vi "ADO Recordset GetString.vi"(0 "ADODB._Recordset":refnum<k7>, 1 "NumRows":i32=-1, 5 "error in (no error)":errorcluster) -> (14 "ADODB._Recordset Out":refnum<k7>, 15 "GetString":string, 19 "error out":errorcluster)   [LabVIEW 2018]
doc: "<FUNCTION>Database Connectivety function.</FUNCTION>\n<DESCRIPTION>Used to get the record set result string</DESCRIPTION>"
panel:
  # "Modified:\n\n2/01 Temp workaround for empty data sets\n2/01 Changed default of NumRows\n5/02 Removed Array From Spreadsheet String, because it trunced the array when a return was inside a db element!"
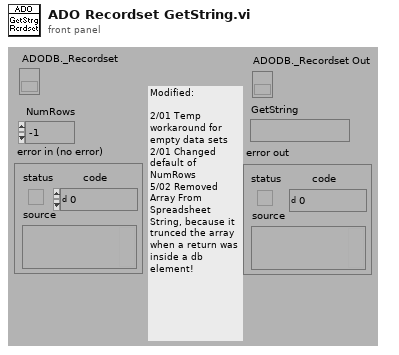
[diagram p1: front panel]
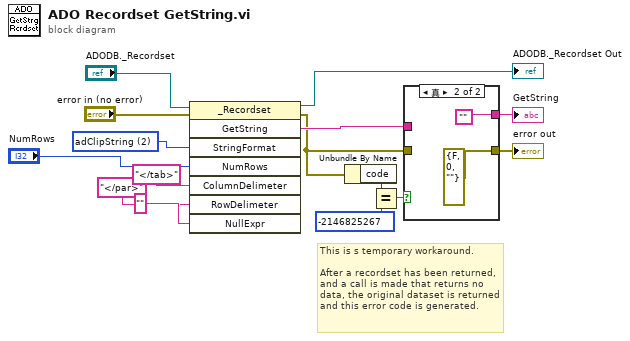
[diagram p0: block diagram]
diagram:
  w14 = 2 items=["adClipString"=2] ("StringFormat")
  # "This is s temporary workaround.\n\nAfter a recordset has been returned, and a call is made that returns no data, the original dataset is returned and this error code is generated."
  n1 = invoke class="_Recordset" method="GetString"(reference="ADODB._Recordset", error in="error in (no error)", "StringFormat"=w14, "NumRows"="NumRows", "ColumnDelimeter"="</tab>", "RowDelimeter"="</par>", "NullExpr"="") -> (reference out=→"ADODB._Recordset Out":refnum<k7>, error out=w1:errorcluster, "GetString"=w3:string)  [unwired: 1 in, 5 out]
  n2 = Unbundle By Name(w1) -> ("code"=w7:i32)
  n3 = Equal?(x=w7, y=-2146825267) -> (x = y?=w5:bool)
  n4 = case shown="真" w5 {
    tunnel: [w17 errorcluster {"status"=FALSE, "code"=0, "source"=""} ("error out")] -> w4
    tunnel: w1 -> [w17 _]
    tunnel: [w16 ""] -> w2
    tunnel: w3 -> [w16 _]
    frame False {
    }
    frame True {
    }
  }
  "error out" <- w4
  "GetString" <- w2
